vi "Autonomous Independent.vi"() -> ()   [LabVIEW 2019]
doc: "This VI is called when autonomous begins, and will automatically be terminated when autonomous ends. You can carry out timed or sensor driven robot movement independently without needing to return to the caller."
uses:
  <vilib>/Rock Robotics/WPI/Utilities/WPI_GetSetVariantRefNum.vi
  <vilib>/Rock Robotics/Network Tables/NT Read String.vi
  <vilib>/Rock Robotics/Network Tables/NT Write Numeric Array.vi
  <vilib>/Rock Robotics/WPI/Ultrasonic/WPI_SonarMB1010AnalogRefNum Registry Get.vi
  <vilib>/Rock Robotics/WPI/Ultrasonic/WPI_SonarMB1010AnalogGetRange.vi
  ultraG.vi
  <vilib>/Rock Robotics/WPI/RobotDrive/WPI_RobotDriveArcadeDrive_Standard(NoSaturation).vi
  <vilib>/Rock Robotics/Network Tables/NT Write Boolean.vi
panel:
  out "Current Movement, for debugging":T1 {"Y Joystick Value" scale=1.0..-1.0; "X Joystick Value" scale=-1.0..1.0}
  in  "Array of robot movements":T2(array[cluster])=[{"X Joystick Value"=0.39393939393939403, "Y Joystick Value"=0.0, "Delay (sec)"=1.0, "Movement Name"="turn"}, {"X Joystick Value"=-0.3737373737373737, "Y Joystick Value"=0.0, "Delay (sec)"=1.0, "Movement Name"="turn back"}] {"Y Joystick Value" scale=1.0..-1.0; "X Joystick Value" scale=-1.0..1.0}
  # "Be sure to right-click and choose Data Operations>>Make Current Value default if you want to save the array values with the VI"
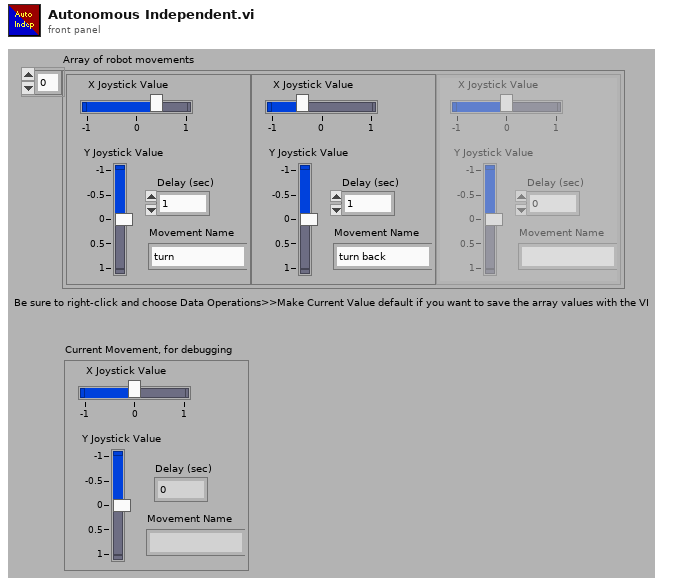
[diagram p1: front panel]
types:
  T1 = cluster{"X Joystick Value":dbl, "Y Joystick Value":dbl, "Delay (sec)":dbl, "Movement Name":string}
  T2 = cluster{"X Joystick Value":dbl, "Y Joystick Value":dbl, "Delay (sec)":dbl, "Movement Name":string}[]
  T3 = typedef "WPI_JoystickDevRef.ctl" = cluster{"Device":T4}
  T4 = typedef "WPI_JoystickDeviceEnum.ctl" = enum16{"USB 0", "USB 1", "USB 2", "USB 3", "USB 4", "USB 5"}
  T5 = typedef "WPI_RobotDriveDevRef.ctl" = cluster{"DevStatus":errorcluster, "Motors[]":T6[], "Square Inputs":bool, "Max Output":dbl}
  T6 = typedef "WPI_MotorControlDeviceRef.ctl" = cluster{"DeviceStatus":errorcluster, "Type":T7, "PWM":cluster{"PWM Channel":T8, "DeadBand":T9}, "CAN":cluster{"Device Number":u8, "SetOutput VI Ref":variant, "GetOutput VI Ref":variant, "Enable VI Ref":variant, "Disable VI Ref":variant, "Data":variant}, "Invert":bool, "DIO PWM":cluster{"PWM \"Enable\" Channel":T8, "DIOChannel":T10, "PWM Rate":dbl}}
  T7 = typedef "WPI_MotorControlType.ctl" = enum16{"PWM", "CAN", "DIO PWM"}
  T8 = typedef "FPGA_DIOPWMChannel.ctl" = enum8{"PWM 0", "PWM 1", "PWM 2", "PWM 3", "PWM 4", "PWM 5", "PWM 6", "PWM 7", "PWM 8", "PWM 9", "PWM MXP 0", "PWM MXP 1", "PWM MXP 2", "PWM MXP 3", "PWM MXP 4", "PWM MXP 5", "PWM MXP 6", "PWM MXP 7", "PWM MXP 8", "PWM MXP 9", "Invalid"}
  T9 = typedef "WPI_PWMDeadband.ctl" = cluster{"Name":string, "maxPositivePwm":i32, "minPositivePwm":i32, "centerPwm":i32, "maxNegativePwm":i32, "minNegativePwm":i32, "angularRange":u16}
  T10 = typedef "FPGA_DIOChannel.ctl" = enum8{"DIO 0", "DIO 1", "DIO 2", "DIO 3", "DIO 4", "DIO 5", "DIO 6", "DIO 7", "DIO 8", "DIO 9", "DIO MXP 0", "DIO MXP 1", "DIO MXP 2", "DIO MXP 3", "DIO MXP 4", "DIO MXP 5", "DIO MXP 6", "DIO MXP 7", "DIO MXP 8", "DIO MXP 9", "DIO MXP 10", "DIO MXP 11", "DIO MXP 12", "DIO MXP 13", "DIO MXP 14", "DIO MXP 15", "SPI Port CS1", "SPI Port CS2", "SPI Port CS3", "SPI Port MISO", "SPI Port MOSI", "Invalid"}
  T11 = typedef "WPI_SonarMB1010AnalogDeviceRef.ctl" = cluster{"AIDeviceRef":T12, "Scaling factor (V/in)":dbl, "Average Bits":u8}
  T12 = typedef "WPI_AnalogChannelDevRef.ctl" = cluster{"DevStatus":errorcluster, "Analog Channel":T13}
  T13 = typedef "FPGA_AIChannel.ctl" = enum8{"AI 0", "AI 1", "AI 2", "AI 3", "AI MXP 0", "AI MXP 1", "AI MXP 2", "AI MXP 3", "Invalid"}
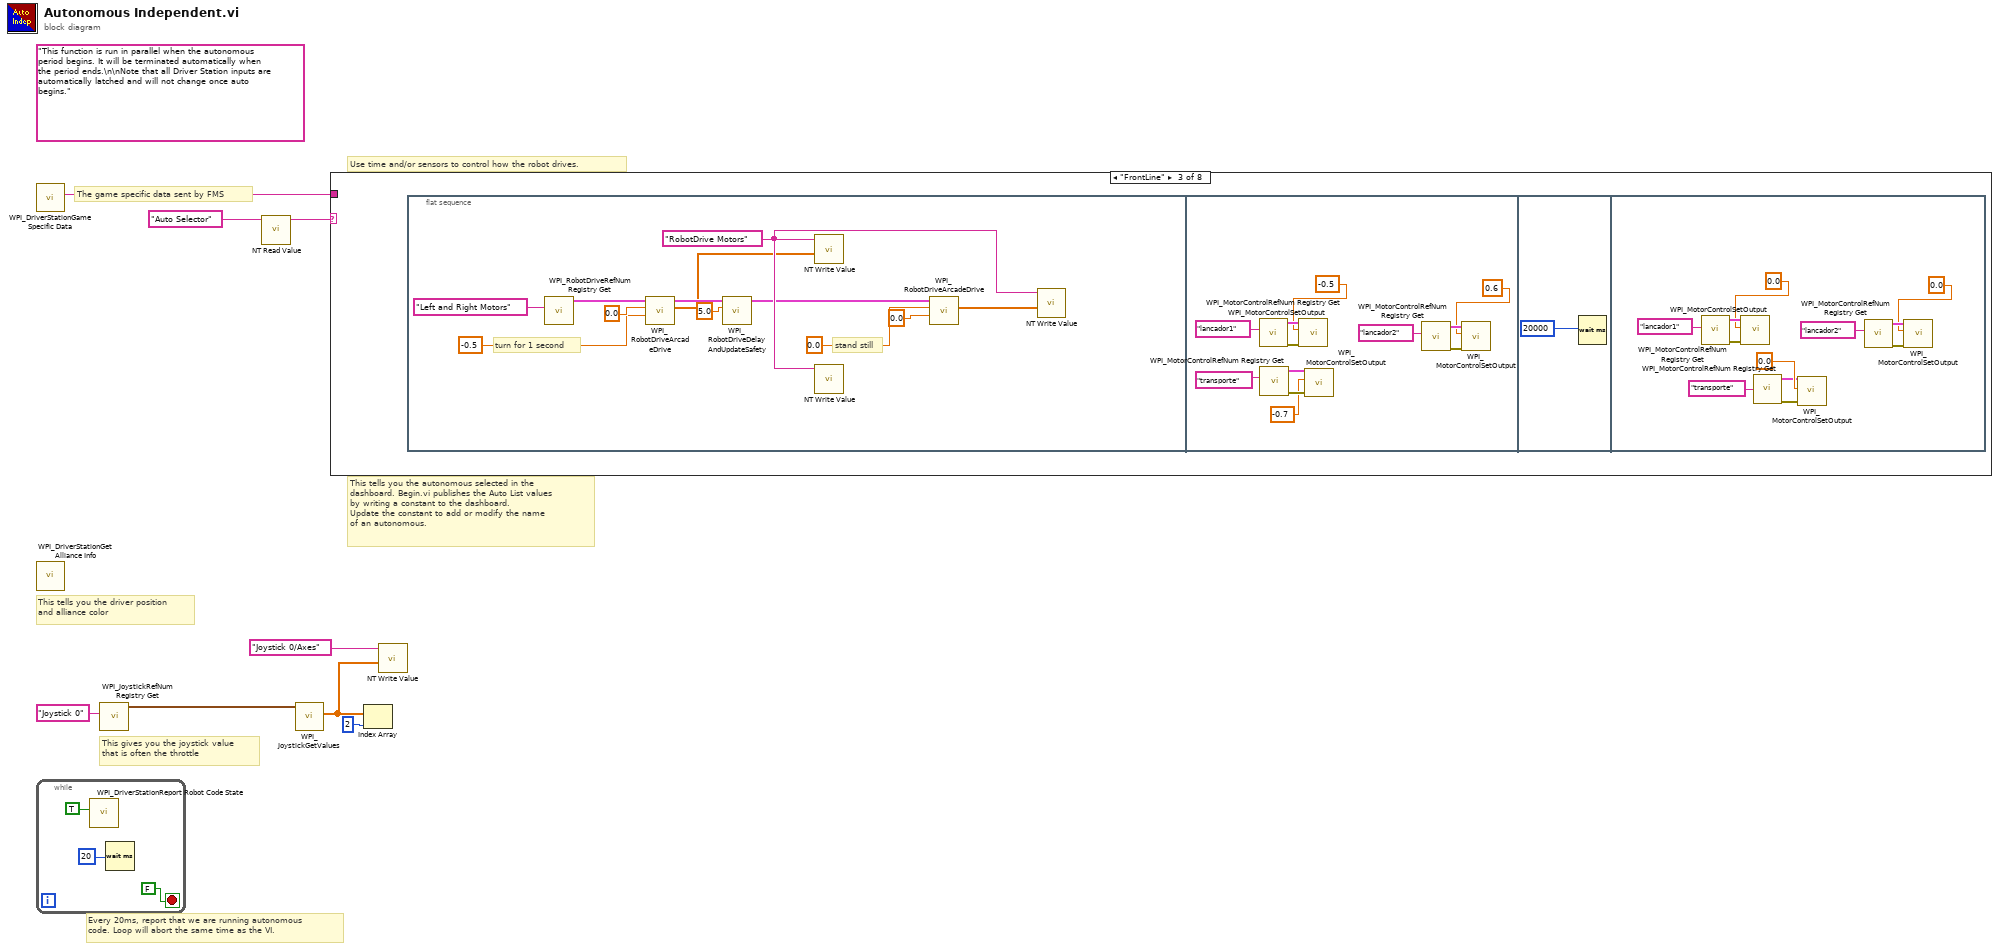
[diagram p0: block diagram]
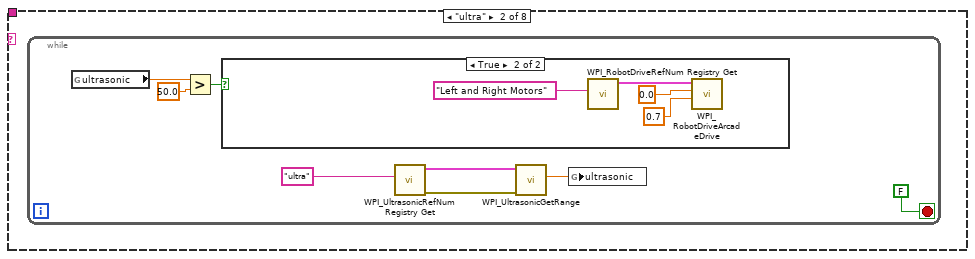
[diagram p3: hidden frame]
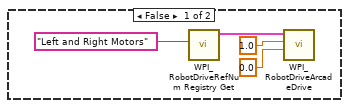
[diagram p4: hidden frame]
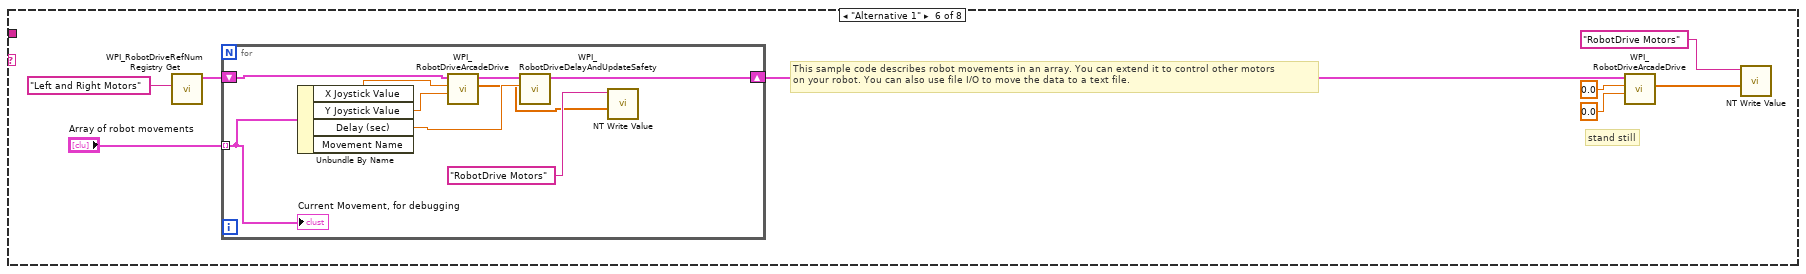
[diagram p7: hidden frame]
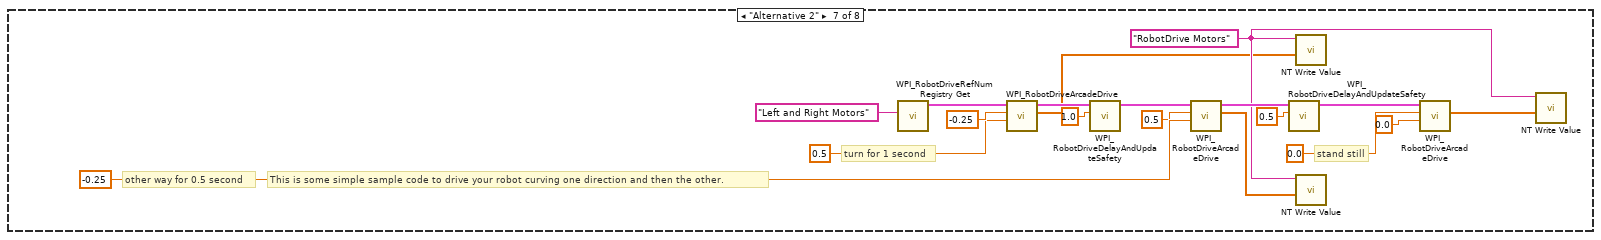
[diagram p8: hidden frame]
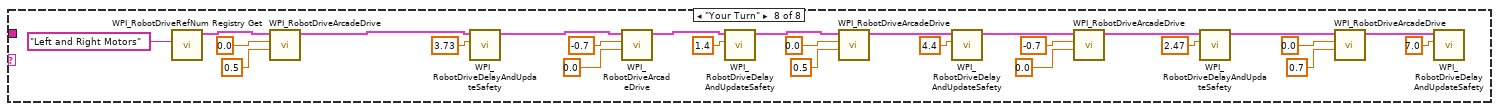
[diagram p9: hidden frame]
diagram:
  (unwired) "This function is run in parallel when the autonomous period begins. It will be terminated automatically when the period ends.\n\nNote that all Driver Station inputs are automatically latched and will not change once auto begins."
  # "The game specific data sent by FMS"
  # "This tells you the autonomous selected in the \ndashboard. Begin.vi publishes the Auto List values\nby writing a constant to the dashboard.\nUpdate the constant to add or modify the name\nof an autonomous."
  # "Every 20ms, report that we are running autonomous\ncode. Loop will abort the same time as the VI."
  # "This gives you the joystick value\nthat is often the throttle"
  # "Use time and/or sensors to control how the robot drives."
  # "This tells you the driver position\nand alliance color"
  n1 = call <vilib>:"WPI_DriverStationGame Specific Data.vi"() -> ("Game Specific Data"=w1:string)  [unwired: 11 in]
  n2 = call <vilib>:"WPI_DriverStationGet Alliance Info.vi"() -> ()  [unwired: 12 out]
  n3 = while {
    stop <- FALSE stop-if-true
    n4 = call <vilib>:"WPI_DriverStationReport Robot Code State.vi"("Autonomous"=TRUE) -> ()  [unwired: 10 in, 1 out]
    n5 = Wait (ms)(milliseconds to wait=u32 20) -> ()  [unwired: 1 out]
  }
  n6 = call <vilib>:"WPI_JoystickRefNum Registry Get.vi"("refnum name"="Joystick 0") -> ("JoystickDevRef"=w7:T3)  [unwired: 1 in, 9 out]
  n7 = call-poly <vilib>:"NT Read Value.vi"("Name"="Auto Selector") -> ("String"=w4:string)  [unwired: 9 in, 1 out]
  n8 = call <vilib>:"WPI_JoystickGetValues.vi"("JoystickDevRef"=w7) -> ("Axes"=w3:dbl[])  [unwired: 6 in, 4 out]
  n9 = case shown="\"FrontLine\"" w4 {
    tunnel: w1 -> [_ _ _ _ _ _ _ _]
    frame Default {
      # "You can put your main auto here, or you can right-click on the case and make any\nother frame be the default case."
      # "This is the frame that will execute if no selection is made, or if it is not recognized"
    }
    frame "ultra" {
      n10 = while {
        stop <- FALSE stop-if-true
        n11 = global read "ultraG.vi" "ultrasonic"() -> (w14:dbl)
        n12 = Greater?(x=w14, y=50.0) -> (0:w13:bool)
        n13 = case shown="True" w13 {
          frame False {
            n14 = call <vilib>:"WPI_RobotDriveRefNum Registry Get.vi"("refnum name"="Left and Right Motors") -> ("RobotDriveDevRef"=w20:T5)  [unwired: 9 in, 1 out]
            n15 = call-poly <vilib>:"WPI_RobotDriveArcadeDrive.vi"("Y axis value"=0.0, "X axis value"=1.0, "RobotDriveDevRef"=w20) -> ()  [unwired: 6 in, 3 out]
          }
          frame True {
            n16 = call <vilib>:"WPI_RobotDriveRefNum Registry Get.vi"("refnum name"="Left and Right Motors") -> ("RobotDriveDevRef"=w24:T5)  [unwired: 9 in, 1 out]
            n17 = call-poly <vilib>:"WPI_RobotDriveArcadeDrive.vi"("Y axis value"=0.7, "X axis value"=0.0, "RobotDriveDevRef"=w24) -> ()  [unwired: 6 in, 3 out]
          }
        }
        n18 = call-poly <vilib>:"WPI_UltrasonicRefNum Registry Get.vi"("refnum name"="ultra") -> ("error out"=w19:errorcluster, "SonarMB1010AnalogDevRef"=w18:T11)  [unwired: 9 in]
        n19 = call-poly <vilib>:"WPI_UltrasonicGetRange.vi"("error in"=w19, "SonarMB1010AnalogDevRef"=w18) -> ("Distance"=w16:dbl)  [unwired: 7 in, 2 out]
        n20 = global write "ultraG.vi" "ultrasonic"(w16) -> ()
      }
    }
    frame "FrontLine" {
      n21 = flat-sequence {
        frame #0 {
          w30 = "RobotDrive Motors" ("Name")
          # "stand still"
          # "turn for 1 second"
          n22 = call <vilib>:"WPI_RobotDriveRefNum Registry Get.vi"("refnum name"="Left and Right Motors") -> ("RobotDriveDevRef"=w39:T5)  [unwired: 1 in, 9 out]
          n23 = call-poly <vilib>:"WPI_RobotDriveArcadeDrive.vi"("Y axis value"=-0.5 ("X axis value"), "X axis value"=0.0, "RobotDriveDevRef"=w39) -> ("Motor Values"=w29:dbl[], "RobotDriveDevRef"=w36:T5)  [unwired: 1 in, 6 out]
          n24 = call <vilib>:"WPI_RobotDriveDelayAndUpdateSafety.vi"("Delay (s)"=5.0, "RobotDriveDevRef"=w36) -> ("RobotDriveDevRef 2"=w28:T5)  [unwired: 8 in, 1 out]
          n25 = call-poly <vilib>:"NT Write Value.vi"("Numeric Array"=w29, "Name"=w30) -> ()  [unwired: 9 in, 1 out]
          n26 = call-poly <vilib>:"NT Write Value.vi"("Name"=w30) -> ()  [unwired: 10 in, 1 out]
          n27 = call-poly <vilib>:"WPI_RobotDriveArcadeDrive.vi"("Y axis value"=0.0 ("X axis value"), "X axis value"=0.0, "RobotDriveDevRef"=w28) -> ("Motor Values"=w31:dbl[])  [unwired: 1 in, 7 out]
          n28 = call-poly <vilib>:"NT Write Value.vi"("Numeric Array"=w31, "Name"=w30) -> ()  [unwired: 9 in, 1 out]
        }
        frame #1 {
          n29 = call <vilib>:"WPI_MotorControlRefNum Registry Get.vi"("refnum name"="lancador1") -> ("error out"=w48:errorcluster, "MotorControlDevRef"=w49:T6)  [unwired: 9 in]
          n30 = call <vilib>:"WPI_MotorControlRefNum Registry Get.vi"("refnum name"="transporte") -> ("error out"=w42:errorcluster, "MotorControlDevRef"=w43:T6)  [unwired: 9 in]
          n31 = call <vilib>:"WPI_MotorControlSetOutput.vi"("error in (no error)"=w48, "Output"=-0.5, "MotorControlDevRef"=w49) -> ()  [unwired: 6 in, 3 out]
          n32 = call <vilib>:"WPI_MotorControlSetOutput.vi"("error in (no error)"=w42, "Output"=-0.7, "MotorControlDevRef"=w43) -> ()  [unwired: 6 in, 3 out]
          n33 = call <vilib>:"WPI_MotorControlRefNum Registry Get.vi"("refnum name"="lancador2") -> ("error out"=w50:errorcluster, "MotorControlDevRef"=w51:T6)  [unwired: 9 in]
          n34 = call <vilib>:"WPI_MotorControlSetOutput.vi"("error in (no error)"=w50, "Output"=0.6, "MotorControlDevRef"=w51) -> ()  [unwired: 6 in, 3 out]
        }
        frame #2 {
          n35 = Wait (ms)(milliseconds to wait=u32 20000) -> ()  [unwired: 1 out]
        }
        frame #3 {
          n36 = call <vilib>:"WPI_MotorControlRefNum Registry Get.vi"("refnum name"="lancador1") -> ("error out"=w61:errorcluster, "MotorControlDevRef"=w62:T6)  [unwired: 9 in]
          n37 = call <vilib>:"WPI_MotorControlSetOutput.vi"("error in (no error)"=w61, "Output"=0.0, "MotorControlDevRef"=w62) -> ()  [unwired: 6 in, 3 out]
          n38 = call <vilib>:"WPI_MotorControlRefNum Registry Get.vi"("refnum name"="transporte") -> ("error out"=w56:errorcluster, "MotorControlDevRef"=w53:T6)  [unwired: 9 in]
          n39 = call <vilib>:"WPI_MotorControlSetOutput.vi"("error in (no error)"=w56, "Output"=0.0, "MotorControlDevRef"=w53) -> ()  [unwired: 6 in, 3 out]
          n40 = call <vilib>:"WPI_MotorControlRefNum Registry Get.vi"("refnum name"="lancador2") -> ("error out"=w63:errorcluster, "MotorControlDevRef"=w64:T6)  [unwired: 9 in]
          n41 = call <vilib>:"WPI_MotorControlSetOutput.vi"("error in (no error)"=w63, "Output"=0.0, "MotorControlDevRef"=w64) -> ()  [unwired: 6 in, 3 out]
        }
      }
    }
    frame "MiddleLine" {
    }
    frame "BackLine" {
    }
    frame "Alternative 1" {
      # "stand still"
      # "This sample code describes robot movements in an array. You can extend it to control other motors\non your robot. You can also use file I/O to move the data to a text file."
      n42 = call <vilib>:"WPI_RobotDriveRefNum Registry Get.vi"("refnum name"="Left and Right Motors") -> ("RobotDriveDevRef"=w71:T5)  [unwired: 1 in, 9 out]
      n43 = for {
        shift-right: [w79] -> w66
        shift-left: w71 -> [w80]
        tunnel: "Array of robot movements" -> [w75] mode=indexing
        n44 = Unbundle By Name(w75) -> ("X Joystick Value"=w78:dbl, "Y Joystick Value"=w77:dbl, "Delay (sec)"=w76:dbl)  [unwired: 1 out]
        n45 = call-poly <vilib>:"WPI_RobotDriveArcadeDrive.vi"("Y axis value"=w77, "X axis value"=w78, "RobotDriveDevRef"=w80) -> ("Motor Values"=w73:dbl[], "RobotDriveDevRef"=w81:T5)  [unwired: 1 in, 6 out]
        n46 = call <vilib>:"WPI_RobotDriveDelayAndUpdateSafety.vi"("Delay (s)"=w76, "RobotDriveDevRef"=w81) -> ("RobotDriveDevRef 2"=w79:T5)  [unwired: 8 in, 1 out]
        n47 = call-poly <vilib>:"NT Write Value.vi"("Numeric Array"=w73, "Name"="RobotDrive Motors") -> ()  [unwired: 9 in, 1 out]
        "Current Movement, for debugging" <- w75
      }
      n48 = call-poly <vilib>:"WPI_RobotDriveArcadeDrive.vi"("Y axis value"=0.0 ("X axis value"), "X axis value"=0.0, "RobotDriveDevRef"=w66) -> ("Motor Values"=w69:dbl[])  [unwired: 1 in, 7 out]
      n49 = call-poly <vilib>:"NT Write Value.vi"("Numeric Array"=w69, "Name"="RobotDrive Motors") -> ()  [unwired: 9 in, 1 out]
    }
    frame "Alternative 2" {
      w83 = "RobotDrive Motors" ("Name")
      # "This is some simple sample code to drive your robot curving one direction and then the other."
      # "stand still"
      # "other way for 0.5 second"
      # "turn for 1 second"
      n50 = call <vilib>:"WPI_RobotDriveRefNum Registry Get.vi"("refnum name"="Left and Right Motors") -> ("RobotDriveDevRef"=w99:T5)  [unwired: 1 in, 9 out]
      n51 = call-poly <vilib>:"WPI_RobotDriveArcadeDrive.vi"("Y axis value"=0.5 ("X axis value"), "X axis value"=-0.25, "RobotDriveDevRef"=w99) -> ("Motor Values"=w82:dbl[], "RobotDriveDevRef"=w92:T5)  [unwired: 1 in, 6 out]
      n52 = call <vilib>:"WPI_RobotDriveDelayAndUpdateSafety.vi"("Delay (s)"=1.0, "RobotDriveDevRef"=w92) -> ("RobotDriveDevRef 2"=w93:T5)  [unwired: 8 in, 1 out]
      n53 = call-poly <vilib>:"WPI_RobotDriveArcadeDrive.vi"("Y axis value"=-0.25 ("X axis value"), "X axis value"=0.5, "RobotDriveDevRef"=w93) -> ("Motor Values"=w84:dbl[], "RobotDriveDevRef"=w94:T5)  [unwired: 1 in, 6 out]
      n54 = call <vilib>:"WPI_RobotDriveDelayAndUpdateSafety.vi"("Delay (s)"=0.5, "RobotDriveDevRef"=w94) -> ("RobotDriveDevRef 2"=w95:T5)  [unwired: 8 in, 1 out]
      n55 = call-poly <vilib>:"NT Write Value.vi"("Numeric Array"=w82, "Name"=w83) -> ()  [unwired: 9 in, 1 out]
      n56 = call-poly <vilib>:"NT Write Value.vi"("Numeric Array"=w84, "Name"=w83) -> ()  [unwired: 9 in, 1 out]
      n57 = call-poly <vilib>:"WPI_RobotDriveArcadeDrive.vi"("Y axis value"=0.0 ("X axis value"), "X axis value"=0.0, "RobotDriveDevRef"=w95) -> ("Motor Values"=w85:dbl[])  [unwired: 1 in, 7 out]
      n58 = call-poly <vilib>:"NT Write Value.vi"("Numeric Array"=w85, "Name"=w83) -> ()  [unwired: 9 in, 1 out]
    }
    frame "Your Turn" {
      n59 = call <vilib>:"WPI_RobotDriveRefNum Registry Get.vi"("refnum name"="Left and Right Motors") -> ("RobotDriveDevRef"=w124:T5)  [unwired: 9 in, 1 out]
      n60 = call-poly <vilib>:"WPI_RobotDriveArcadeDrive.vi"("Y axis value"=0.5, "X axis value"=0.0, "RobotDriveDevRef"=w124) -> ("RobotDriveDevRef"=w121:T5)  [unwired: 6 in, 2 out]
      n61 = call <vilib>:"WPI_RobotDriveDelayAndUpdateSafety.vi"("Delay (s)"=3.73, "RobotDriveDevRef"=w121) -> ("RobotDriveDevRef 2"=w118:T5)  [unwired: 8 in, 1 out]
      n62 = call-poly <vilib>:"WPI_RobotDriveArcadeDrive.vi"("Y axis value"=0.0, "X axis value"=-0.7, "RobotDriveDevRef"=w118) -> ("RobotDriveDevRef"=w117:T5)  [unwired: 6 in, 2 out]
      n63 = call <vilib>:"WPI_RobotDriveDelayAndUpdateSafety.vi"("Delay (s)"=1.4, "RobotDriveDevRef"=w117) -> ("RobotDriveDevRef 2"=w114:T5)  [unwired: 8 in, 1 out]
      n64 = call-poly <vilib>:"WPI_RobotDriveArcadeDrive.vi"("Y axis value"=0.5, "X axis value"=0.0, "RobotDriveDevRef"=w114) -> ("RobotDriveDevRef"=w112:T5)  [unwired: 6 in, 2 out]
      n65 = call <vilib>:"WPI_RobotDriveDelayAndUpdateSafety.vi"("Delay (s)"=4.4, "RobotDriveDevRef"=w112) -> ("RobotDriveDevRef 2"=w109:T5)  [unwired: 8 in, 1 out]
      n66 = call-poly <vilib>:"WPI_RobotDriveArcadeDrive.vi"("Y axis value"=0.0, "X axis value"=-0.7, "RobotDriveDevRef"=w109) -> ("RobotDriveDevRef"=w108:T5)  [unwired: 6 in, 2 out]
      n67 = call <vilib>:"WPI_RobotDriveDelayAndUpdateSafety.vi"("Delay (s)"=2.47, "RobotDriveDevRef"=w108) -> ("RobotDriveDevRef 2"=w104:T5)  [unwired: 8 in, 1 out]
      n68 = call-poly <vilib>:"WPI_RobotDriveArcadeDrive.vi"("Y axis value"=0.7, "X axis value"=0.0, "RobotDriveDevRef"=w104) -> ("RobotDriveDevRef"=w103:T5)  [unwired: 6 in, 2 out]
      n69 = call <vilib>:"WPI_RobotDriveDelayAndUpdateSafety.vi"("Delay (s)"=7.0, "RobotDriveDevRef"=w103) -> ()  [unwired: 8 in, 2 out]
    }
  }
  n70 = Index Array(array=w3, index=2) -> ()  [unwired: 1 out]
  n71 = call-poly <vilib>:"NT Write Value.vi"("Numeric Array"=w3, "Name"="Joystick 0/Axes") -> ()  [unwired: 9 in, 1 out]
